vi "NitrateCalculator(SubVI).vi"() -> (0 "A'- Graph":cluster{dbl[], dbl[]}[](graph)=[{[210.47, 211.013, 211.556, 212.099, 212.642, 213.185, 213.728, 214.271, 214.814, 215.357, 215.9, 216.443, 216.986, 217.529, 218.072, 218.615, 219.158, 219.701, 220.244, 220.787, 221.33, 221.873, 222.416, 222.959, 223.502, 224.045, 224.588, 225.131, 225.674, 226.217, 226.76, 227.303, 227.846, 228.389, 228.932, 229.475, 230.018, 230.561, 231.104, 231.647, 232.19, 232.733, 233.276, 233.819, 234.362, 234.905, 235.448, 235.991, 236.534, 237.077, 237.62, 238.163, 238.706, 239.249, 239.792, 240.335, 240.878, 241.421, 241.964, 242.507, 243.05, 243.593, 244.136, 244.679, 245.222, 245.765, 246.308, 246.851, 247.394, 247.937, 248.48, 249.023, 249.566, 250.109, 250.652, 251.195, 251.738, 252.281, 252.824, 253.367, 253.91, 254.453, 254.996, 255.539, 256.082, 256.625, 257.168, 257.711, 258.254, 258.797, 259.34, 259.883], [0.12793016694096082, 0.1327881561828641, 0.13898634561838696, 0.1259197207741436, 0.14132650024267335, 0.14734372113403094, 0.1485442487837778, 0.14751986962096558, 0.13775057031586085, 0.1454257108067617, 0.13827874574091015, 0.1380955602332684, 0.13280214091499964, 0.13096155295962347, 0.1242263335792905, 0.1200317395047893, 0.11520703411258498, 0.10969549971555982, 0.10694233961076889, 0.10205574991791058, 0.09580016806982122, 0.09167882996708734, 0.08624690930416284, 0.08168334522252357, 0.0789249659761026, 0.07423828091165904, 0.06873855259983944, 0.06612583621347973, 0.06228574814736767, 0.056930857187937944, 0.05331141850375127, 0.049396798883806, 0.04725985884383318, 0.042960378591267154, 0.040558634335614574, 0.038548841416862094, 0.03383136521287019, 0.031853948056984105, 0.02956088014857819, 0.027222379512650333, 0.02497238017948171, 0.022053860485673114, 0.02039542923280995, 0.01879516854143684, 0.016254370606103935, 0.015144480862862991, 0.013534765266055699, 0.012169541069378806, 0.01021984544175458, 0.008561791484343755, 0.008019447576661586, 0.006251714332178242, 0.0055858813703053, 0.004428072374523385, 0.0033942758849625923, 0.0031852781299558422, 0.0026522707441254765, 0.0024666851934537033, 0.0015639696080979272, 0.0005833772835681486, 0.0006126350464351532, 0.0013427440658959052, -0.0001526640434080166, -0.00018534269449400128, -0.0008475009717322837, -0.0006159477395225686, -0.0012976525297084872, -0.0013704938482608702, -0.001798765017845805, -0.0027720616232884314, -0.002333163582774802, -0.0006534404274150182, -0.0011629877379098984, -0.0027525829787817795, -0.00016639630496898049, -0.0004977867659968762, -0.0013551881915035838, -0.0010474447563982889, -0.000676610158729499, -0.0005184402556335553, -0.0012932934214892246, -0.0008002296314189829, -0.001006272911124815, -9.314949136806912e-05, 0.0003192583376444662, -0.00022800478420321665, 0.0003585188526099983, 0.0020169373032707903, 0.0017243828096380077, 0.001655229240884793, 0.002495498904283519, 0.002648662191671046]}], 1 "ENo3- Graph":cluster{dbl[], dbl[]}[](graph)=[{[210.47, 211.013, 211.556, 212.099, 212.642, 213.185, 213.728, 214.271, 214.814, 215.357, 215.9, 216.443, 216.986, 217.529, 218.072, 218.615, 219.158, 219.701, 220.244, 220.787, 221.33, 221.873, 222.416, 222.959, 223.502, 224.045, 224.588, 225.131, 225.674, 226.217, 226.76, 227.303, 227.846, 228.389, 228.932, 229.475, 230.018, 230.561, 231.104, 231.647, 232.19, 232.733, 233.276, 233.819, 234.362, 234.905, 235.448, 235.991, 236.534, 237.077, 237.62, 238.163, 238.706, 239.249, 239.792, 240.335, 240.878, 241.421, 241.964, 242.507, 243.05, 243.593, 244.136, 244.679, 245.222, 245.765, 246.308, 246.851, 247.394, 247.937, 248.48, 249.023, 249.566, 250.109, 250.652, 251.195, 251.738, 252.281, 252.824, 253.367, 253.91, 254.453, 254.996, 255.539, 256.082, 256.625, 257.168, 257.711, 258.254, 258.797, 259.34, 259.883], [294533.0127801271, 298085.5275880313, 343627.90959666116, 376974.47849339014, 386689.4510497263, 408487.361468496, 402337.995919341, 394279.2626230384, 384148.70174255007, 400065.5053294645, 382821.7589663287, 381729.96302631096, 360204.34492696734, 344168.1761747931, 338547.79019137163, 319190.9477478034, 302790.09884812176, 282791.62400064373, 275816.1391723025, 255944.0213948449, 235254.35629028594, 221131.94352582796, 207125.4044684568, 187249.85984661555, 175797.55053965125, 161037.56628618063, 148122.20799419747, 139190.41799350036, 131246.02246379605, 117807.92525407567, 104692.42425921683, 95048.85917176834, 85301.43961733059, 79807.3512786411, 72998.70960192374, 66030.96910237371, 58007.034950494846, 52190.91337484809, 48103.63900398817, 41426.41235694945, 39643.69339279932, 32675.55408020507, 30180.301544036793, 26077.982058174846, 21827.834165794342, 20317.512601786377, 17200.08873168833, 15225.53896286287, 12672.119927733758, 10510.81741692185, 8868.612370915853, 7402.308578565035, 7497.783663214231, 5843.7467508738355, 2592.4790276671915, 3972.3290964164526, 2801.6242550079305, 2194.681099032995, 483.755084946024, 925.3260306661116, 368.7216063147762, 656.4562628975337, -310.2759697380701, -348.22870243873723, -825.7001809816267, -2448.7077528786954, -753.0208161604538, -1900.9160404506808, -2978.370140188913, -2381.9749647347458, -2825.2299308214206, -632.5350510303439, 344.6192065771905, -2197.6730977680554, 2222.006114722468, -46.74799630302776, -1784.5052107769725, -11.357589657642048, -1.7334389454220873, 685.1118545455417, -1056.1490174616833, -714.5991484163018, -156.31996144296522, -83.38814015497948, -1462.8189953991298, -612.5489805889721, 839.9819289346627, 2059.4630435447557, 1295.6187847181666, -94.77195505370497, 2304.784809174573, 2473.487218805406]}], 2 "Absorbancs Graph":cluster{dbl[], dbl[]}[](graph)=[{[210.47, 211.013, 211.556, 212.099, 212.642, 213.185, 213.728, 214.271, 214.814, 215.357, 215.9, 216.443, 216.986, 217.529, 218.072, 218.615, 219.158, 219.701, 220.244, 220.787, 221.33, 221.873, 222.416, 222.959, 223.502, 224.045, 224.588, 225.131, 225.674, 226.217, 226.76, 227.303, 227.846, 228.389, 228.932, 229.475, 230.018, 230.561, 231.104, 231.647, 232.19, 232.733, 233.276, 233.819, 234.362, 234.905, 235.448, 235.991, 236.534, 237.077, 237.62, 238.163, 238.706, 239.249, 239.792, 240.335, 240.878, 241.421, 241.964, 242.507, 243.05, 243.593, 244.136, 244.679, 245.222, 245.765, 246.308, 246.851, 247.394, 247.937, 248.48, 249.023, 249.566, 250.109, 250.652, 251.195, 251.738, 252.281, 252.824, 253.367, 253.91, 254.453, 254.996, 255.539, 256.082, 256.625, 257.168, 257.711, 258.254, 258.797, 259.34, 259.883], [0.859775678286318, 0.8194318156296146, 0.7895662441158913, 0.7653583418970374, 0.7134020372603199, 0.6674930001591154, 0.6169042198464642, 0.5666594591614739, 0.5127610913357338, 0.4760432747417854, 0.43179210618385533, 0.39546521483677954, 0.35704563080021307, 0.3204937163802063, 0.2943543872023645, 0.2644968000756883, 0.23727151168709026, 0.21506292164762564, 0.19582373256481655, 0.17509578429484746, 0.15778012766612576, 0.14182714481381176, 0.12762613288942176, 0.11359011007339652, 0.10311798710231297, 0.0919810390323458, 0.08407740857125809, 0.07520310011257239, 0.06894533118889845, 0.06156116409513224, 0.054721465538073055, 0.04951119044573565, 0.04379079748078188, 0.040522877073344524, 0.03583986731239025, 0.03120271181313547, 0.02776368982361145, 0.024890944782316078, 0.021970298789674186, 0.019046917639680402, 0.017650784209329966, 0.014430138184920574, 0.012660635378348474, 0.010678518980179588, 0.00996203492854495, 0.00865803175790969, 0.007123137178893124, 0.006459897966245347, 0.005454774486390257, 0.004673433507016052, 0.00317899640396703, 0.002978638971630067, 0.0032063812554244536, 0.0025374593715086283, 0.0010371917010740805, 0.0013682683081331706, 0.0012338025827769855, 0.00044231588608750066, 0.0006576235447054053, 0.0003592638366740966, 3.86590865093725e-05, -5.462381588621987e-05, -0.00043697341233217557, 0.00028768565388054973, -0.0005029989692543549, -0.0003836845555745434, -2.1769830005107654e-05, -8.158566931395356e-05, -0.0012657429248070888, -0.0009881653780830016, -0.0006206450872670022, -0.0008460195763415369, -0.0008440728182035687, -0.0008541442548795249, 0.0003212150192799558, -0.00016824964081266214, -0.0006849404823446592, 0.0004342318774892516, 0.00025692780195036777, 0.00010544427557851802, 0.00044687325757008026, -0.00017318641138520594, -4.097812470797019e-05, -8.4835930852626e-05, -0.00032452033611190395, -0.0006147450240710922, 0.00011997159689319109, -0.00015409533396294056, 0.0006683040427777585, 0.00014999181500151976, 0.0010128166761367956, 0.0012425823150642307]}, {[210.47, 211.013, 211.556, 212.099, 212.642, 213.185, 213.728, 214.271, 214.814, 215.357, 215.9, 216.443, 216.986, 217.529, 218.072, 218.615, 219.158, 219.701, 220.244, 220.787, 221.33, 221.873, 222.416, 222.959, 223.502, 224.045, 224.588, 225.131, 225.674, 226.217, 226.76, 227.303, 227.846, 228.389, 228.932, 229.475, 230.018, 230.561, 231.104, 231.647, 232.19, 232.733, 233.276, 233.819, 234.362, 234.905, 235.448, 235.991, 236.534, 237.077, 237.62, 238.163, 238.706, 239.249, 239.792, 240.335, 240.878, 241.421, 241.964, 242.507, 243.05, 243.593, 244.136, 244.679, 245.222, 245.765, 246.308, 246.851, 247.394, 247.937, 248.48, 249.023, 249.566, 250.109, 250.652, 251.195, 251.738, 252.281, 252.824, 253.367, 253.91, 254.453, 254.996, 255.539, 256.082, 256.625, 257.168, 257.711, 258.254, 258.797, 259.34, 259.883], [0.801341170479744, 0.7542734132237421, 0.6980568093186122, 0.65420605249337, 0.591680060881281, 0.5299625392926228, 0.47702592078260647, 0.4255234062398998, 0.3711647669162868, 0.3228829251218208, 0.2827599748503002, 0.2434409059716668, 0.2119311833930049, 0.1798378791449536, 0.15402672866461736, 0.13094215234558915, 0.10931855345881111, 0.09491646684250218, 0.07742521143320874, 0.06462685612767415, 0.05592972771866379, 0.04553833460727783, 0.03699743050859016, 0.031488515184952236, 0.025748999955385175, 0.020904706258801094, 0.018642890097352365, 0.013432623513669001, 0.010553223074843139, 0.009115474310373156, 0.008106302412446732, 0.00717074031072442, 0.005744777726777169, 0.004893684096016718, 0.0031711878437890757, 0.0015769760381964641, 0.0017569164268725172, 0.001484919073282149, 0.00034167784506089136, 0.00042709614687959363, -0.00019894237181035043, -0.0002881289314805198, -0.0009673652556734837, -0.0011091138604324736, 0.000146281936226407, -0.0005078123746470216, -0.0006453921276296619, -0.00040921704838469547, -0.00025853371894282023, -5.8841081421987657e-05, -0.0008455489737523095, -0.0003666006559215444, -0.0001741794938470015, -9.572694367300863e-05, -0.00013418443402012092, -0.0004342119920670712, -2.785591609676813e-05, -0.0005634379748792259, 0.0004540623443782983, -5.8901234707184336e-05, -0.00013105680029032452, -0.0003600499082511144, -0.0003055170322483515, 0.00045608059860526365, -0.00013473988615758312, 0.0007354698007963102, 0.00032433285193672265, 0.0007906108278793178, 7.605421447198432e-05, 8.534654960939622e-05, 0.0006625762183634851, -0.0005709729804337961, -0.0010150816524892026, 0.0001368035849654524, -0.000687954722901625, -0.00014905489719789847, 0.00011942950940802693, 0.000443837174362572, 0.00026005063494623573, -0.00020446941719183195, 0.000928426415228837, 0.000149226286241394, 2.9499413362117644e-05, -4.747285768441287e-05, 0.00033451056635025456, -0.00033948938772015297, -0.00025802686603175473, -0.0010796627525889724, 8.508559467040183e-05, 0.00019199329640829516, -2.422754560728671e-05, 0.00012878794244869374]}, {[210.47, 211.013, 211.556, 212.099, 212.642, 213.185, 213.728, 214.271, 214.814, 215.357, 215.9, 216.443, 216.986, 217.529, 218.072, 218.615, 219.158, 219.701, 220.244, 220.787, 221.33, 221.873, 222.416, 222.959, 223.502, 224.045, 224.588, 225.131, 225.674, 226.217, 226.76, 227.303, 227.846, 228.389, 228.932, 229.475, 230.018, 230.561, 231.104, 231.647, 232.19, 232.733, 233.276, 233.819, 234.362, 234.905, 235.448, 235.991, 236.534, 237.077, 237.62, 238.163, 238.706, 239.249, 239.792, 240.335, 240.878, 241.421, 241.964, 242.507, 243.05, 243.593, 244.136, 244.679, 245.222, 245.765, 246.308, 246.851, 247.394, 247.937, 248.48, 249.023, 249.566, 250.109, 250.652, 251.195, 251.738, 252.281, 252.824, 253.367, 253.91, 254.453, 254.996, 255.539, 256.082, 256.625, 257.168, 257.711, 258.254, 258.797, 259.34, 259.883], [0.8349250299196103, 0.7985659782220785, 0.7554294716845671, 0.7039073271955195, 0.6643155846589284, 0.6159979981150474, 0.5705818180332749, 0.5241666942013795, 0.4664351446159479, 0.4314871898047554, 0.3889092668584453, 0.35397500896861966, 0.32082659223672977, 0.29058708622423546, 0.26100520078520395, 0.23636505571931815, 0.212374355658777, 0.1941007847601965, 0.17582536275176977, 0.15957915032302233, 0.14560551256364115, 0.13224949336973374, 0.11922368957919263, 0.1097629242038428, 0.10189705539077057, 0.0928971760093605, 0.08538635126587726, 0.07812652408738596, 0.07171836378664848, 0.06508217851129808, 0.060563676829728776, 0.0558150422512567, 0.052404168918151785, 0.04734459073599655, 0.043400995888894185, 0.03996295459186795, 0.03540756730509166, 0.033186749038576574, 0.029867698307559296, 0.027606079350583596, 0.024793568873241023, 0.02179476713041542, 0.019525144001637858, 0.01779689632707871, 0.016386094716066633, 0.014686993002350365, 0.012953061761290088, 0.011800535044244484, 0.009986607793191861, 0.008508683009597853, 0.007255921855678818, 0.005920522311633751, 0.005428452139574033, 0.004341510976025073, 0.003272882804573607, 0.002792275615607423, 0.002627046818162858, 0.001956247104735409, 0.001975511612610885, 0.0005299670100274712, 0.0004937405679766166, 0.0010159557259308144, -0.00043008610603853525, 0.00022898969989317702, -0.0009699640550975969, 5.282040887574779e-05, -0.0010025972441931735, -0.0006509174041809049, -0.0017295119228779299, -0.0026943110513844987, -0.0017292772649578902, -0.0011740793412730113, -0.0020890149910946926, -0.0026277233640298464, -0.0007945791770674893, -0.0006339544985643902, -0.0012460337713899386, -0.0006416045454584116, -0.0004387120217184681, -0.0007055787813360359, -0.00044316594100983486, -0.0006635248767982091, -0.0009792362292916634, -0.00013667933511483932, 0.0006261275336703967, -0.0005395860806047259, 0.00012159334130024124, 0.0010251084460011217, 0.0018025827427642638, 0.001831767211735412, 0.0024732113092995472, 0.002767192854815498]}], 3 "[NO3] Linear fit":dbl=0.39513021806615695 format="%#_3g")   [LabVIEW 2019]
uses:
  Global.vi
panel:
  in  "Path Length":dbl=33.85 format="%#_13g"
  in  "[NO3-]":dbl=4.5e-05 caption="Known Nitrate Concentration"
  in  "S(TS)":dbl=33.66 caption="Sample Water Salinity" format="%#_13g"
  in  "S(KN)":dbl=33.85 caption="Calibration Salinity" format="%#_13g"
  in  "T(KN)":dbl=21.0 caption="Calibration Temp Zero Nitrate" format="%#_13g"
  in  "S(Norm)":dbl=35.0 caption="Calibration Salinity" format="%#_13g"
  in  "T(TS)":dbl=20.0 caption="Test Sample Sea Water Temp" format="%#_13g"
  in  "T(ZN)":dbl=19.3 caption="Calibration Temp Zero Nitrate" format="%#_13g"
  in  "S(ZN)":dbl=36.052 caption="Zero Nitrate Sea Water  Salinity" format="%#_13g"
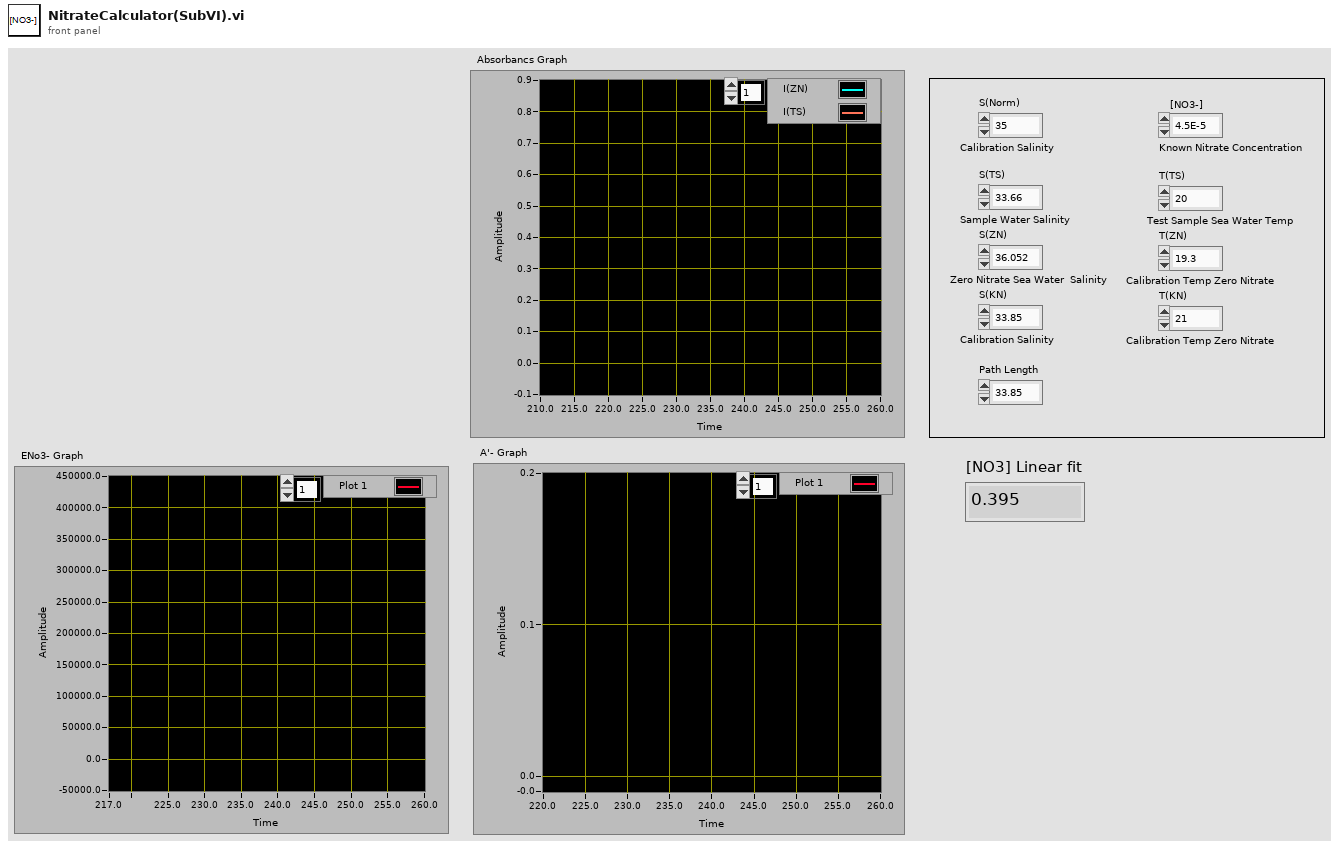
[diagram p1: front panel]
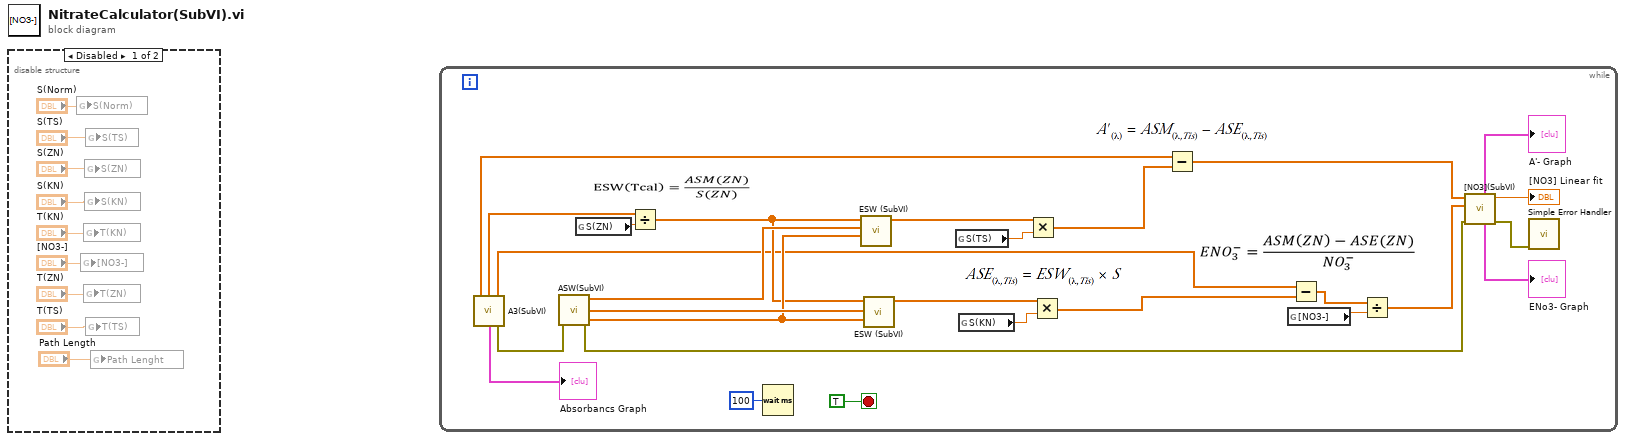
[diagram p0: block diagram]
diagram:
  n1 = disable-structure shown="Disabled" {
    frame Disabled {
      n2 = global write "Global.vi" "S(Norm)"("S(Norm)") -> ()
      n3 = global write "Global.vi" "[NO3-]"("[NO3-]") -> ()
      n4 = global write "Global.vi" "T(KN)"("T(KN)") -> ()
      n5 = global write "Global.vi" "T(ZN)"("T(ZN)") -> ()
      n6 = global write "Global.vi" "S(ZN)"("S(ZN)") -> ()
      n7 = global write "Global.vi" "S(KN)"("S(KN)") -> ()
      n8 = global write "Global.vi" "S(TS)"("S(TS)") -> ()
      n9 = global write "Global.vi" "T(TS)"("T(TS)") -> ()
      n10 = global write "Global.vi" "Path Lenght"("Path Length") -> ()
    }
    frame Enabled {
    }
  }
  n11 = while {
    stop <- TRUE stop-if-true
    n12 = call "A3(SubVI).vi"() -> ("error out"=w13:errorcluster, "A(ZN)"=w18:dbl[], "A(KN)"=w20:dbl[], "A(TS)"=w19:dbl[], "Absorbancs Graph"=→"Absorbancs Graph":cluster{dbl[], dbl[]}[])  [unwired: 7 in]
    n13 = call "ASW(SubVI).vi"("error in (no error)"=w13) -> ("error out"=w35:errorcluster, "ASW(TS)"=w31:dbl[], "ASW(KN)"=w33:dbl[], "ASW(ZN)"=w32:dbl[])  [unwired: 7 in]
    n14 = global read "Global.vi" "S(ZN)"() -> (w26:dbl)
    n15 = Divide(x=w18, y=w26) -> (x/y=w22:dbl[])
    n16 = Wait (ms)(milliseconds to wait=u32 100) -> ()  [unwired: 1 out]
    n17 = call "ESW (SubVI).vi"("ASW(ZN)"=w32, "ASW(KN)"=w31, "ESW(in)"=w22) -> ("ESW(out)"=w21:dbl[])  [unwired: 8 in]
    n18 = call "ESW (SubVI).vi"("ASW(ZN)"=w32, "ASW(KN)"=w33, "ESW(in)"=w22) -> ("ESW(out)"=w23:dbl[])  [unwired: 8 in]
    n19 = global read "Global.vi" "S(TS)"() -> (w25:dbl)
    n20 = global read "Global.vi" "S(KN)"() -> (w24:dbl)
    n21 = Multiply(x=w21, y=w25) -> (x*y=w28:dbl[])
    n22 = Multiply(x=w23, y=w24) -> (x*y=w29:dbl[])
    n23 = Subtract(x=w19, y=w28) -> (x-y=w12:dbl[])
    n24 = global read "Global.vi" "[NO3-]"() -> (w27:dbl)
    n25 = Subtract(x=w20, y=w29) -> (x-y=w30:dbl[])
    n26 = Divide(x=w30, y=w27) -> (x/y=w16:dbl[])
    n27 = call "[NO3](SubVI).vi"("error in (no error)"=w35, "ENo3-"=w16, "A'"=w12) -> ("error out"=w15:errorcluster, "[NO3]"=→"[NO3] Linear fit":dbl, "ENo3- Graph"=→"ENo3- Graph":cluster{dbl[], dbl[]}[], "A'- Graph"=→"A'- Graph":cluster{dbl[], dbl[]}[])  [unwired: 5 in]
    n28 = call <vilib>:"Simple Error Handler.vi"("error in (no error)"=w15) -> ()  [unwired: 4 in, 5 out]
  }
